vi "MakeScanFilename.vi"(9 "Program":string[][](table), 10 "index (row)":i32, 11 "Sample directory":path) -> (2 "path":path)   [LabVIEW 2013]
uses:
  controls/ProgramColumn.ctl
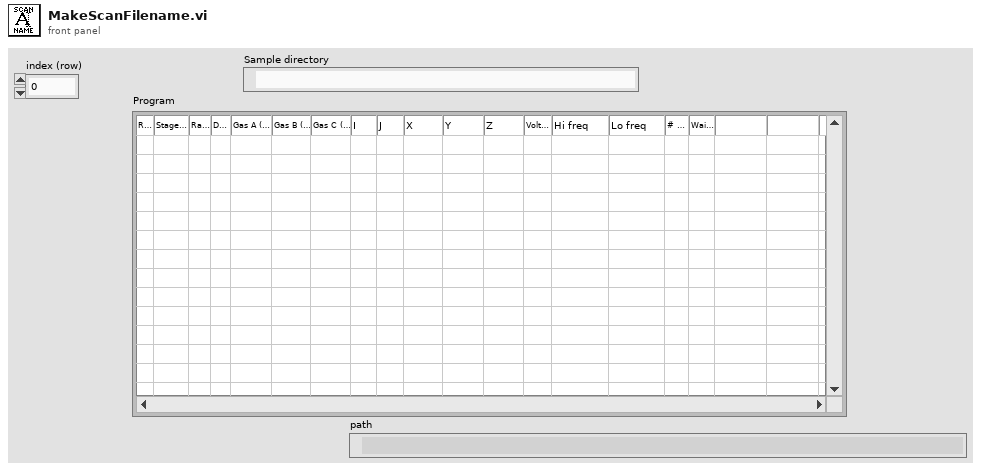
[diagram p1: front panel]
types:
  T1 = typedef "ProgramColumn.ctl" = enum16{"Run Number", "Stage Temperature", "Ramp Rate", "Wait", "Gas A", "Gas B", "Gas C", "Row index I", "Column index J", "X position", "Y position", "Z position", "Voltage", "Highest frequency", "Lowest frequency", "Number of freq pts", "Delay", "Move this step?", "bias(V)"}
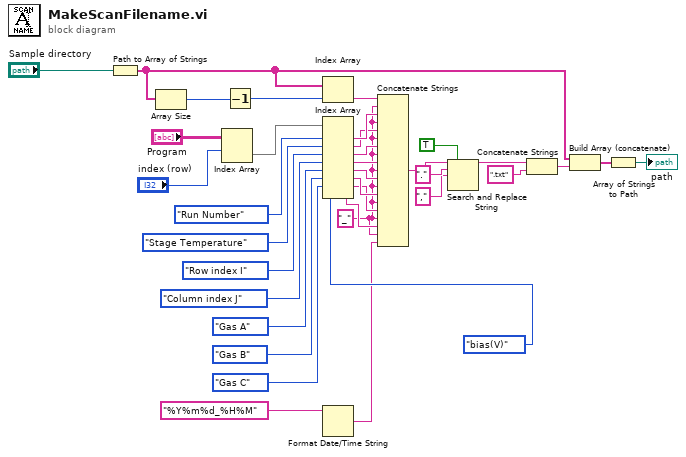
[diagram p0: block diagram]
diagram:
  w2 = "_"
  n1 = Path to Array of Strings(0:"Sample directory") -> (2:w31:string[])  [unwired: 1 out]
  n2 = Array Size(array=w31) -> (size(s)=w35:i32)
  n3 = Index Array(array="Program", index (row)="index (row)") -> (element=w24:string[])  [unwired: 1 in]
  n4 = Decrement(x=w35) -> (x-1=w34:i32)
  n5 = Index Array(array=w31, index=w34) -> (element=w23:string)
  n6 = Index Array(array=w24, index #1=ProgramColumn."Run Number" ("Enum"), index #2=ProgramColumn."Stage Temperature" ("Enum"), index #3=ProgramColumn."Row index I" ("Enum"), index #4=ProgramColumn."Column index J" ("Enum"), index #5=ProgramColumn."Gas A" ("Enum"), index #6=ProgramColumn."Gas B" ("Enum"), index #7=ProgramColumn."Gas C" ("Enum"), index #8=ProgramColumn."bias(V)" ("Enum")) -> (element #1=w22:string, element #2=w21:string, element #3=w20:string, element #4=w19:string, element #5=w10:string, element #6=w9:string, element #7=w8:string, element #8=w3:string)
  n7 = Format Date/Time String(time format string (%c)="%Y%m%d_%H%M") -> (date/time string=w1:string)  [unwired: 2 in]
  n8 = Concatenate Strings(w23, w2, w22, w2, w21, w2, w20, w2, w19, w2, w10, w2, w9, w2, w8, w2, w3, w2, w1) -> (w11:string)
  n9 = Search and Replace String(replace all?=TRUE ("replace all? (F)"), input string=w11, search string=".", replace string="," ("replace string (\"\")")) -> (result string=w5:string)  [unwired: 4 in, 3 out]
  n10 = Concatenate Strings(w5, ".txt" ("string")) -> (w6:string)
  n11 = Build Array (concatenate)(w31, w6) -> (w30:string[])
  n12 = Array of Strings to Path(0:w30) -> (2:→"path":path)  [unwired: 1 in]
